vi "addImgToTree.vi"(5 "Bildunterschrifft":string, 6 "Numeric":i32, 8 "error in (no error)":errorcluster, 9 "Elternobjekt-Tag":string, 10 "selected path":path, 11 "TreeControl in":refnum<vi>) -> (0 "error out":errorcluster)   [LabVIEW 2013, in "DataCreation.lvlib"]
uses:
  DataCreation.lvlib
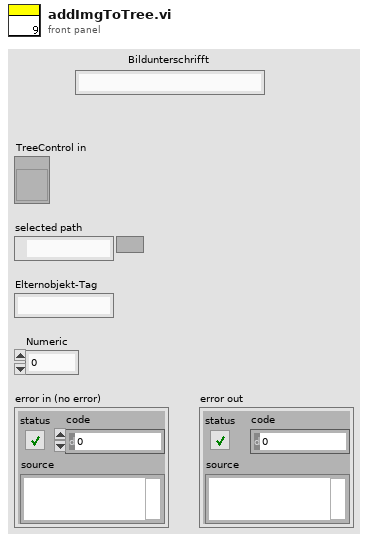
[diagram p1: front panel]
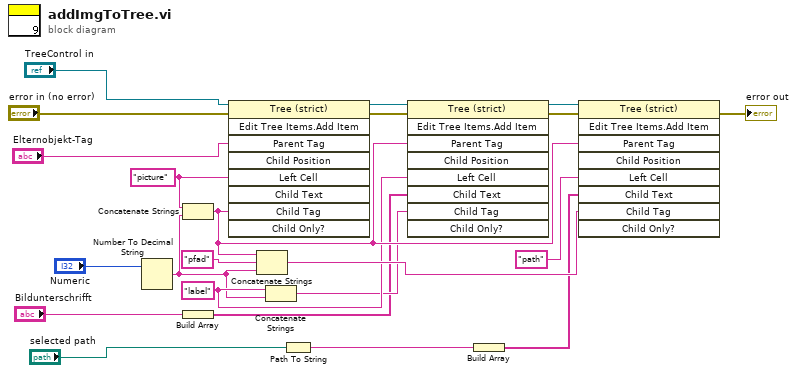
[diagram p0: block diagram]
diagram:
  w12 = "label" ("Left Cell String")
  w2 = "picture" ("Left Cell String")
  n1 = Number To Decimal String(number="Numeric") -> (decimal integer string=w11:string)  [unwired: 1 in]
  n2 = Concatenate Strings(w2, w11) -> (w13:string)
  n3 = Build Array("Bildunterschrifft") -> (w5:string[])
  n4 = invoke class="Tree (strict)" method="Edit Tree Items.Add Item"(reference="TreeControl in", error in="error in (no error)", "Parent Tag"="Elternobjekt-Tag", "Left Cell"=w2, "Child Tag"=w13) -> (reference out=w8:refnum<vi>, error out=w4:errorcluster)  [unwired: 4 in, 7 out]
  n5 = Concatenate Strings(w13, "pfad", w11) -> (w15:string)
  n6 = Concatenate Strings(w12, w11) -> (w10:string)
  n7 = Path To String(path="selected path") -> (string=w6:string)
  n8 = invoke class="Tree (strict)" method="Edit Tree Items.Add Item"(reference=w8, error in=w4, "Parent Tag"=w13, "Left Cell"=w12, "Child Text"=w5, "Child Tag"=w10) -> (reference out=w7:refnum<vi>, error out=w3:errorcluster)  [unwired: 3 in, 7 out]
  n9 = Build Array(w6) -> (w9:string[])
  n10 = invoke class="Tree (strict)" method="Edit Tree Items.Add Item"(reference=w7, error in=w3, "Parent Tag"=w13, "Left Cell"="path" ("Left Cell String"), "Child Text"=w9, "Child Tag"=w15) -> (error out=→"error out":errorcluster)  [unwired: 3 in, 8 out]
